vi "Open XL Application.vi"(8 "error in":errorcluster) -> (0 "error out":errorcluster, 2 "Excel.Workbooks":refnum<k7>, 3 "Excel._Application":refnum<k7>)   [LabVIEW 2017]
panel:
  in  "Excel._Application 2":refnum<k7>
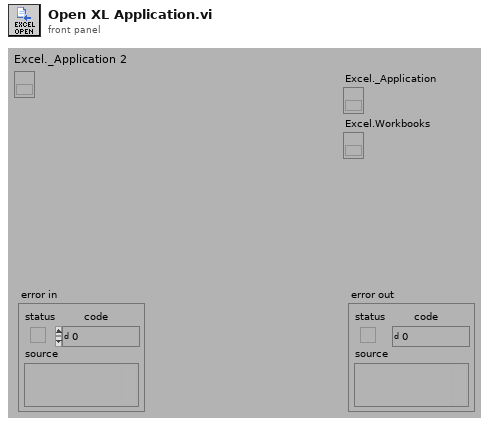
[diagram p1: front panel]
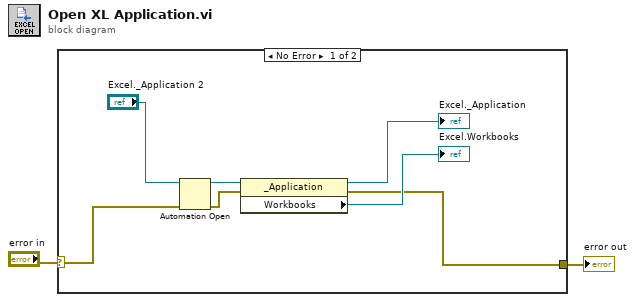
[diagram p0: block diagram]
diagram:
  n1 = case shown="No Error" "error in" {
    selector: "error in" -> [w9 w10]
    tunnel: [w4 w10] -> w1
    frame No Error {
      n2 = Automation Open(error in (no error)=w9, Automation Refnum="Excel._Application 2") -> (Automation Refnum=w6:refnum<k7>, error out=w8:errorcluster)  [unwired: 2 out]
      n3 = property class="_Application"(reference=w6, error in=w8) -> (reference out=→"Excel._Application":refnum<k7>, error out=w4:errorcluster, "Workbooks"=→"Excel.Workbooks":refnum<k7>)
    }
    frame Error {
    }
  }
  "error out" <- w1
